vi "Alter Macro.vi"(7 "Action":enum16{"Add", "Insert", "Modify", "Delete"}(ring)=enum."Delete", 10 "Steps in":T1[](array[typedef])) -> (2 "Steps out":T1[](array[typedef]))   [LabVIEW 2020, in "MacroAssert.lvlib"]
doc: "Higher level VI for performing a number of actions on a profile. Takes <B>Action</B> as an input and executes code that performs that action."
uses:
  MacroAssert.lvlib
  CTLs/Step V3.ctl
  CTLs/Step Type V3.ctl
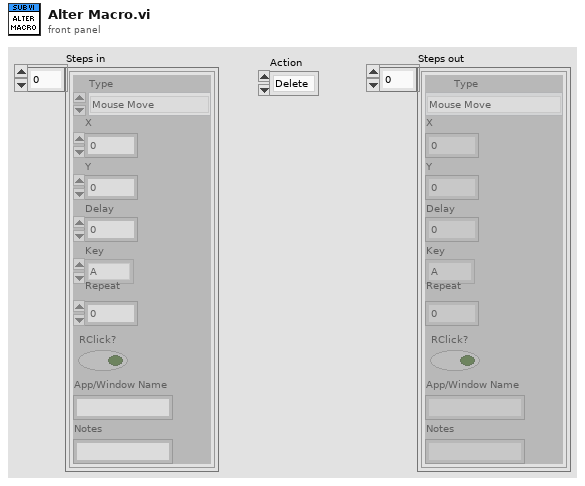
[diagram p1: front panel]
types:
  T1 = typedef "MacroAssert.lvlib/Step V3.ctl" = cluster{"Type":T2, "X":i32, "Y":i32, "Delay":i32, "Key":u8, "Repeat":i32, "RClick?":bool, "App/Window Name":string, "Notes":string}
  T2 = typedef "MacroAssert.lvlib/Step Type V3.ctl" = enum16{"Mouse Move", "Mouse Click", "Key Press", "Wait", "Mouse Down", "Mouse Up", "Key Down", "Key Up", "Run Application", "Maximize Window", "Restore Window", "Minimize Window", "Close Window", "Bring Window to Front", "Send Window to Back"}
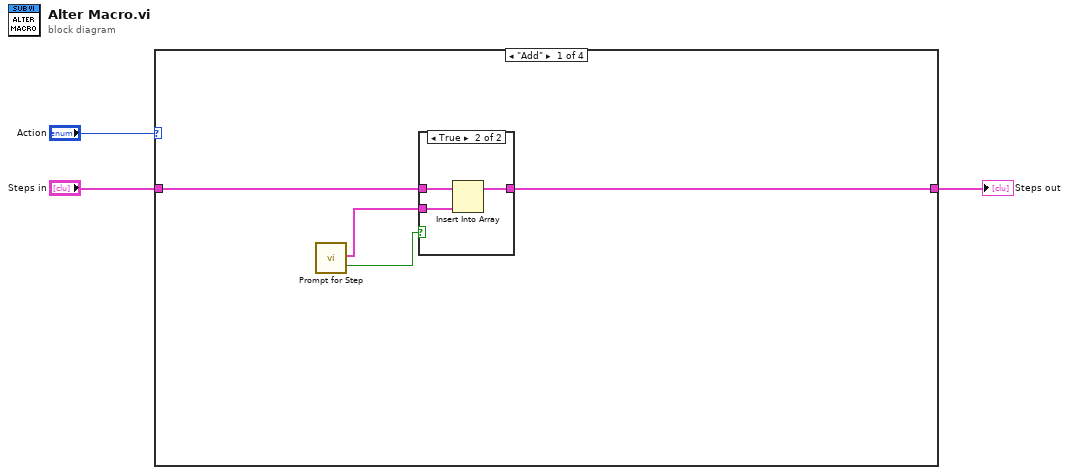
[diagram p0: block diagram]
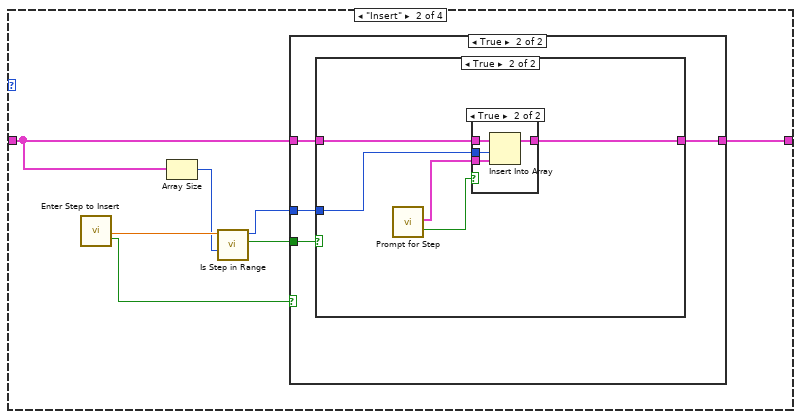
[diagram p3: hidden frame]
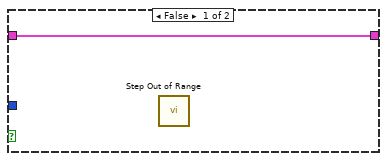
[diagram p5: hidden frame]
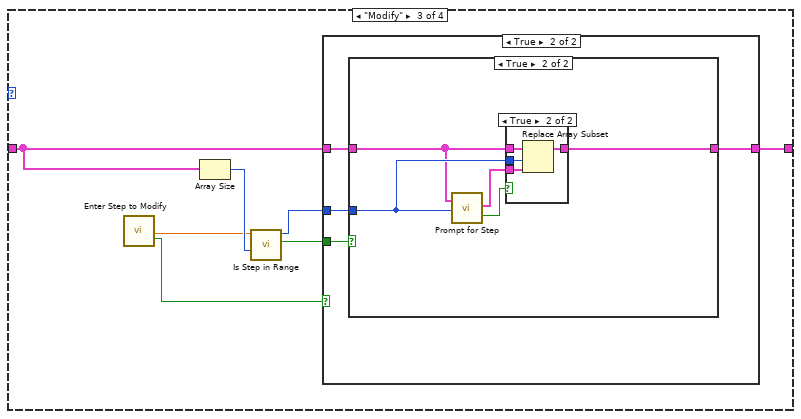
[diagram p7: hidden frame]
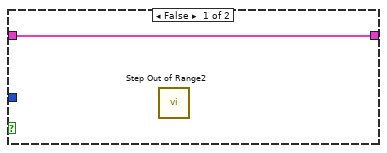
[diagram p9: hidden frame]
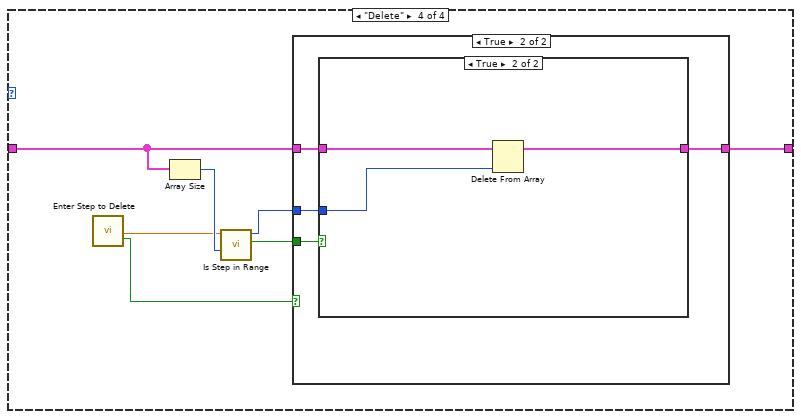
[diagram p11: hidden frame]
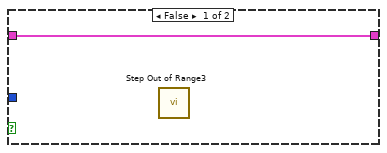
[diagram p13: hidden frame]
diagram:
  n1 = case shown="\"Add\"" "Action" {
    tunnel: "Steps in" -> [w6 w13 w36 w59]
    tunnel: [w5 w12 w35 w58] -> w1
    frame "Add" {
      n2 = call "Prompt for Step.vi"() -> ("New Data Out"=w7:T1, "OK?"=w4:bool)  [unwired: 17 in, 1 out]
      n3 = case shown="True" w4 {
        tunnel: w7 -> [_ w11]
        tunnel: w6 -> [w8 w10]
        tunnel: [w8 w9] -> w5
        frame False {
        }
        frame True {
          n4 = Insert Into Array(array=w10, new element=w11) -> (w9:T1[])  [unwired: 1 in]
        }
      }
    }
    frame "Insert" {
      n5 = call "Enter Step to Insert"() -> ("Step"=w17:dbl, "OK"=w18:bool)  [unwired: 17 in, 1 out]
      n6 = Array Size(array=w13) -> (size(s)=w16:i32)
      n7 = call "Is Step in Range.vi"("Array Size"=w16, "Chosen Step"=w17) -> ("In Range?"=w15:bool, "Index out"=w14:i32)  [unwired: 8 in]
      n8 = case shown="True" w18 {
        tunnel: w15 -> [_ w23]
        tunnel: w14 -> [_ w22]
        tunnel: w13 -> [w19 w21]
        tunnel: [w19 w20] -> w12
        frame False {
        }
        frame True {
          n9 = case shown="True" w23 {
            tunnel: w22 -> [_ w29]
            tunnel: w21 -> [w24 w27]
            tunnel: [w24 w26] -> w20
            frame False {
              n10 = call "Step Out of Range"() -> ()  [unwired: 10 in, 2 out]
            }
            frame True {
              n11 = call "Prompt for Step.vi"() -> ("New Data Out"=w28:T1, "OK?"=w25:bool)  [unwired: 17 in, 1 out]
              n12 = case shown="True" w25 {
                tunnel: w29 -> [_ w34]
                tunnel: w28 -> [_ w33]
                tunnel: w27 -> [w30 w32]
                tunnel: [w30 w31] -> w26
                frame False {
                }
                frame True {
                  n13 = Insert Into Array(array=w32, index=w34, new element=w33) -> (w31:T1[])
                }
              }
            }
          }
        }
      }
    }
    frame "Modify" {
      n14 = call "Enter Step to Modify"() -> ("Step"=w38:dbl, "OK"=w37:bool)  [unwired: 17 in, 1 out]
      n15 = Array Size(array=w36) -> (size(s)=w41:i32)
      n16 = call "Is Step in Range.vi"("Array Size"=w41, "Chosen Step"=w38) -> ("In Range?"=w40:bool, "Index out"=w39:i32)  [unwired: 8 in]
      n17 = case shown="True" w37 {
        tunnel: w40 -> [_ w46]
        tunnel: w39 -> [_ w45]
        tunnel: w36 -> [w42 w44]
        tunnel: [w42 w43] -> w35
        frame False {
        }
        frame True {
          n18 = case shown="True" w46 {
            tunnel: w45 -> [_ w52]
            tunnel: w44 -> [w47 w49]
            tunnel: [w47 w50] -> w43
            frame False {
              n19 = call "Step Out of Range2"() -> ()  [unwired: 10 in, 2 out]
            }
            frame True {
              n20 = call "Prompt for Step.vi"("Steps"=w49, "Index"=w52) -> ("New Data Out"=w51:T1, "OK?"=w48:bool)  [unwired: 15 in, 1 out]
              n21 = case shown="True" w48 {
                tunnel: w52 -> [_ w57]
                tunnel: w51 -> [_ w56]
                tunnel: [w53 w55] -> w50
                tunnel: w49 -> [w53 w54]
                frame False {
                }
                frame True {
                  n22 = Replace Array Subset(array=w54, new element=w56, index=w57) -> (w55:T1[])
                }
              }
            }
          }
        }
      }
    }
    frame "Delete" {
      n23 = call "Enter Step to Delete"() -> ("Step"=w61:dbl, "OK"=w60:bool)  [unwired: 17 in, 1 out]
      n24 = Array Size(array=w59) -> (size(s)=w64:i32)
      n25 = call "Is Step in Range.vi"("Array Size"=w64, "Chosen Step"=w61) -> ("In Range?"=w63:bool, "Index out"=w62:i32)  [unwired: 8 in]
      n26 = case shown="True" w60 {
        tunnel: w63 -> [_ w69]
        tunnel: w62 -> [_ w68]
        tunnel: w59 -> [w65 w67]
        tunnel: [w65 w66] -> w58
        frame False {
        }
        frame True {
          n27 = case shown="True" w69 {
            tunnel: w68 -> [_ w73]
            tunnel: w67 -> [w70 w72]
            tunnel: [w70 w71] -> w66
            frame False {
              n28 = call "Step Out of Range3"() -> ()  [unwired: 10 in, 2 out]
            }
            frame True {
              n29 = Delete From Array(array=w72, index=w73) -> (array with subset deleted=w71:T1[])  [unwired: 1 in, 1 out]
            }
          }
        }
      }
    }
  }
  "Steps out" <- w1
